vi "executePlay.vi"(8 "error in (no error)":errorcluster, 11 "Game in":refnum<class "Game.lvclass">) -> (0 "error out":errorcluster, 3 "Game out":refnum<class "Game.lvclass">)   [LabVIEW 2018, in "Game.lvclass"]
uses:
  Game.lvclass
  Game.lvclass/Game.ctl
  Team_class/Team.lvclass/Team.ctl
  Playbook_class/Playbook.lvclass/Playbook.ctl
  TestPlay_class/TestPlay.lvclass/TestPlay.ctl
  Robot_class/Robot.lvclass/Robot.ctl
  Robot_class/Read role.vi
  Playbook_class/Read defensive_plays.vi
  TestPlay_class/Read Roles.vi
  Playbook_class/Read offensive_plays.vi
  Playbook_class/Read keeper_plays.vi
  Read Utilities.lvclass.vi
  Read AllyRef.vi
  Read Playbook.vi
  Team_class/Read RobotRef.vi
  Team_class/Read KeeperPlay.vi
  Team_class/Read OffensivePlay.vi
  Team_class/Read DefensivePlay.vi
  Team_class/Write RobotRef.vi
  Write AllyRef.vi
  Ally_class/Ally.lvclass
  C:/Users/nicolas.oliveira/roboime/SSL_AI/Team_class/Team.lvclass
  Utilities_class/Utilities.lvclass
  Playbook_class/Playbook.lvclass
  Robot_class/Robot.lvclass
  Play_class/Play.lvclass
  TestPlay_class/TestPlay.lvclass
  TestRole_class/TestRole.lvclass
  Role_class/Role.lvclass
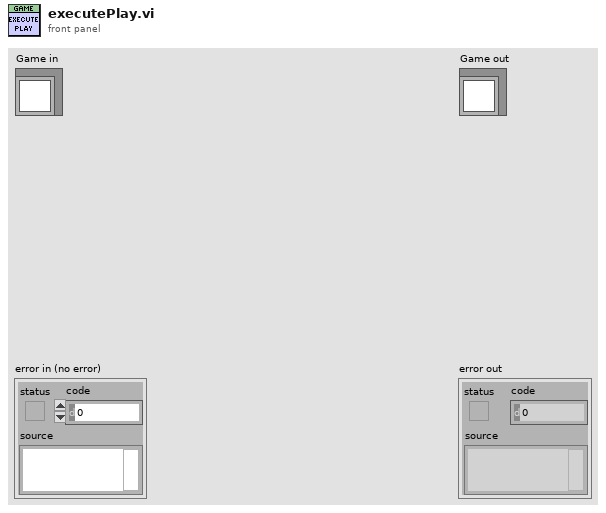
[diagram p1: front panel]
types:
  T1 = typedef "KeeperPlay.ctl" = enum16{"NormalGame", "Halt", "Timeout", "PenaltyEnemy", "TestPlay"}
  T2 = typedef "OffensivePlay.ctl" = enum16{"TestPlay", "PreparePenaltyAlly", "KickPenaltyAlly", "PrepareKickoffAlly", "PrepareKickoffEnemy", "IndirectEnemy", "DirectEnemy", "NormalGame", "NormalGameEnemyPossesion", "DirectKick", "Pass", "Halt", "Timeout", "PenaltyEnemy"}
  T3 = typedef "DefensivePlay.ctl" = enum16{"TestPlay", "Default", "Duelist", "Halt", "Timeout", "PenaltyEnemy", "PenaltyAlly"}
  T4 = cluster{"Play":refnum<class "Play.lvclass">, "TestPlay":refnum<class "TestPlay.lvclass">}
  T5 = typedef "roles.ctl" = enum16{"Role", "TestRole"}
  T6 = cluster{"TestRole":refnum<class "TestRole.lvclass">, "Role":refnum<class "Role.lvclass">}
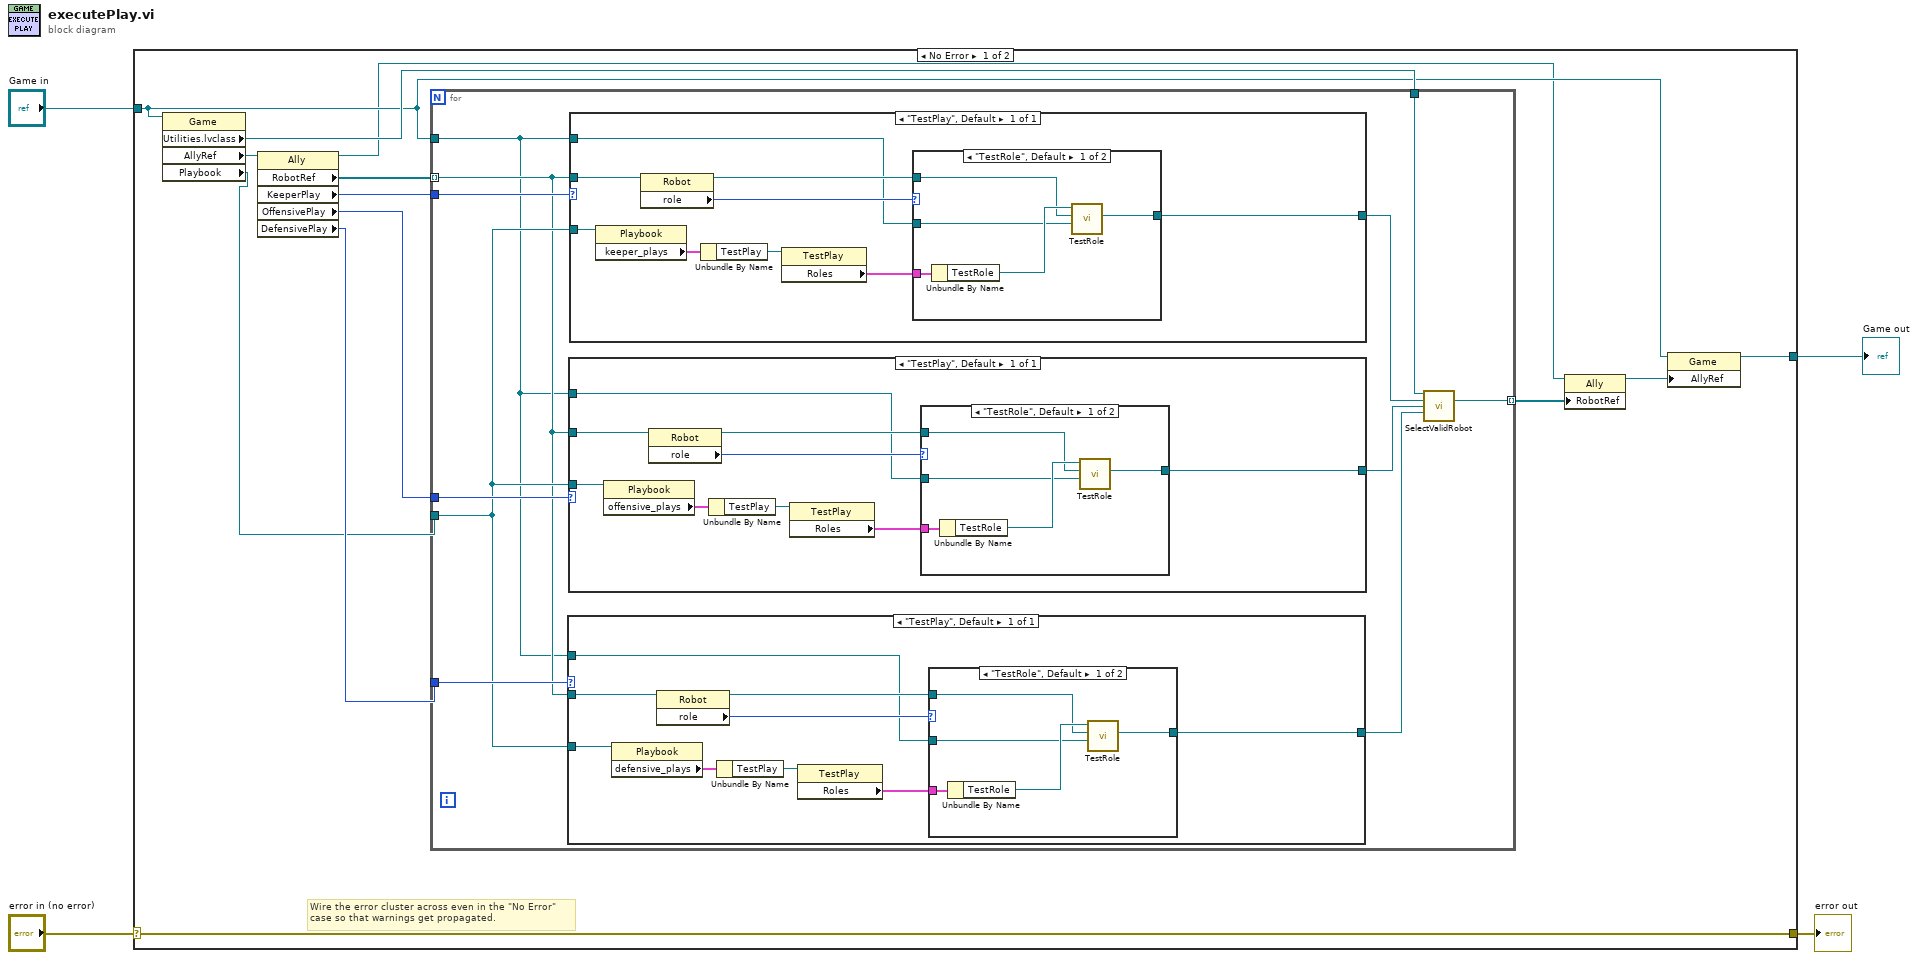
[diagram p0: block diagram]
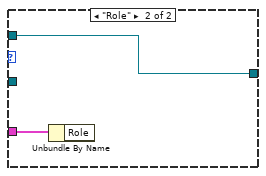
[diagram p2: hidden frame]
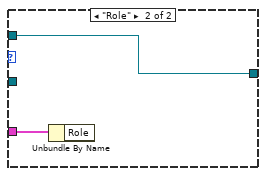
[diagram p3: hidden frame]
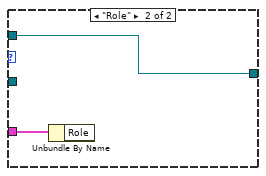
[diagram p4: hidden frame]
diagram:
  n1 = case shown="No Error" "error in (no error)" {
    selector: "error in (no error)" -> [w17 w78]
    tunnel: [w17 w78] -> w3
    tunnel: [w5 w77] -> w1
    tunnel: "Game in" -> [w9 w77]
    frame No Error {
      # "Wire the error cluster across even in the \"No Error\"\ncase so that warnings get propagated."
      n2 = property class="Game"(reference=w9) -> ("Utilities.lvclass"=w10:refnum<class "Utilities.lvclass">, "AllyRef"=w16:refnum<class "Ally.lvclass">, "Playbook"=w11:refnum<class "Playbook.lvclass">)  [unwired: 1 in, 2 out]
      n3 = property class="Ally"(reference=w16) -> (reference out=w8:refnum<class "Ally.lvclass">, "RobotRef"=w15:refnum<class "Robot.lvclass">[], "KeeperPlay"=w14:T1, "OffensivePlay"=w13:T2, "DefensivePlay"=w12:T3)  [unwired: 1 in, 1 out]
      n4 = for {
        tunnel: w15 -> [w22] mode=indexing
        tunnel: w14 -> [w28]
        tunnel: w13 -> [w27]
        tunnel: w12 -> [w26]
        tunnel: w11 -> [w25]
        tunnel: w9 -> [w21]
        tunnel: w10 -> [w23]
        tunnel: [w18] -> w7 mode=indexing
        n5 = case shown="\"TestPlay\", Default" w26 {
          tunnel: w25 -> [w32]
          tunnel: w21 -> [w31]
          tunnel: w22 -> [w30]
          tunnel: [w29] -> w19
          frame "TestPlay", Default {
            n6 = property class="Playbook"(reference=w32) -> ("defensive_plays"=w37:T4)  [unwired: 1 in, 2 out]
            n7 = property class="Robot"(reference=w30) -> (reference out=w33:refnum<class "Robot.lvclass">, "role"=w35:T5)  [unwired: 1 in, 1 out]
            n8 = Unbundle By Name(w37) -> ("TestPlay"=w36:refnum<class "TestPlay.lvclass">)
            n9 = property class="TestPlay"(reference=w36) -> ("Roles"=w34:T6)  [unwired: 1 in, 2 out]
            n10 = case shown="\"TestRole\", Default" w35 {
              tunnel: w34 -> [w42 w44]
              tunnel: w33 -> [w40 w43]
              tunnel: w31 -> [w39 _]
              tunnel: [w38 w43] -> w29
              frame "TestRole", Default {
                n11 = Unbundle By Name(w42) -> ("TestRole"=w41:refnum<class "TestRole.lvclass">)
                n12 = call-dynamic "TestRole.vi"("Game in"=w39, "Robot in"=w40, "TestRole in"=w41) -> ("Robot out"=w38:refnum<class "Robot.lvclass">)  [unwired: 5 in, 3 out]
              }
              frame "Role" {
                n13 = Unbundle By Name(w44) -> ()  [unwired: 1 out]
              }
            }
          }
        }
        n14 = case shown="\"TestPlay\", Default" w27 {
          tunnel: w25 -> [w48]
          tunnel: w22 -> [w47]
          tunnel: w21 -> [w46]
          tunnel: [w45] -> w20
          frame "TestPlay", Default {
            n15 = property class="Playbook"(reference=w48) -> ("offensive_plays"=w49:T4)  [unwired: 1 in, 2 out]
            n16 = property class="Robot"(reference=w47) -> (reference out=w53:refnum<class "Robot.lvclass">, "role"=w51:T5)  [unwired: 1 in, 1 out]
            n17 = Unbundle By Name(w49) -> ("TestPlay"=w50:refnum<class "TestPlay.lvclass">)
            n18 = property class="TestPlay"(reference=w50) -> ("Roles"=w52:T6)  [unwired: 1 in, 2 out]
            n19 = case shown="\"TestRole\", Default" w51 {
              tunnel: w52 -> [w58 w60]
              tunnel: w53 -> [w56 w59]
              tunnel: w46 -> [w55 _]
              tunnel: [w54 w59] -> w45
              frame "TestRole", Default {
                n20 = Unbundle By Name(w58) -> ("TestRole"=w57:refnum<class "TestRole.lvclass">)
                n21 = call-dynamic "TestRole.vi"("Game in"=w55, "Robot in"=w56, "TestRole in"=w57) -> ("Robot out"=w54:refnum<class "Robot.lvclass">)  [unwired: 5 in, 3 out]
              }
              frame "Role" {
                n22 = Unbundle By Name(w60) -> ()  [unwired: 1 out]
              }
            }
          }
        }
        n23 = case shown="\"TestPlay\", Default" w28 {
          tunnel: w25 -> [w69]
          tunnel: w22 -> [w66]
          tunnel: w21 -> [w62]
          tunnel: [w61] -> w24
          frame "TestPlay", Default {
            n24 = property class="Playbook"(reference=w69) -> ("keeper_plays"=w68:T4)  [unwired: 1 in, 2 out]
            n25 = property class="Robot"(reference=w66) -> (reference out=w63:refnum<class "Robot.lvclass">, "role"=w65:T5)  [unwired: 1 in, 1 out]
            n26 = Unbundle By Name(w68) -> ("TestPlay"=w67:refnum<class "TestPlay.lvclass">)
            n27 = property class="TestPlay"(reference=w67) -> ("Roles"=w64:T6)  [unwired: 1 in, 2 out]
            n28 = case shown="\"TestRole\", Default" w65 {
              tunnel: w64 -> [w74 w76]
              tunnel: w63 -> [w72 w75]
              tunnel: w62 -> [w71 _]
              tunnel: [w70 w75] -> w61
              frame "TestRole", Default {
                n29 = Unbundle By Name(w74) -> ("TestRole"=w73:refnum<class "TestRole.lvclass">)
                n30 = call-dynamic "TestRole.vi"("Game in"=w71, "Robot in"=w72, "TestRole in"=w73) -> ("Robot out"=w70:refnum<class "Robot.lvclass">)  [unwired: 5 in, 3 out]
              }
              frame "Role" {
                n31 = Unbundle By Name(w76) -> ()  [unwired: 1 out]
              }
            }
          }
        }
        n32 = call-dynamic "SelectValidRobot.vi"("Utilities in"=w23, "Robot 1"=w24, "Robot 2"=w20, "Robot 3"=w19) -> ("Robot out"=w18:refnum<class "Robot.lvclass">)  [unwired: 9 in, 2 out]
      }
      n33 = property class="Ally"(reference=w8, "RobotRef"=w7) -> (reference out=w6:refnum<class "Ally.lvclass">)  [unwired: 1 in, 1 out]
      n34 = property class="Game"(reference=w9, "AllyRef"=w6) -> (reference out=w5:refnum<class "Game.lvclass">)  [unwired: 1 in, 1 out]
    }
    frame Error {
    }
  }
  "error out" <- w3
  "Game out" <- w1
